vi "Acq 3.5 FPGA.vi"() -> ()   [LabVIEW 2021]
uses:
  <vilib>/rvi/Emulation/niFpgaGetClockAttributes.vi
  <vilib>/rvi/Emulation/niFpgaSctlEmulationGetInTimedLoop.vi
  <vilib>/rvi/Emulation/niFpgaEmulationReportErrorSimple.vi
  <vilib>/rvi/eio/common/nirviEmuTemplateMethod_errors.vi
  <vilib>/rvi/interface/RandomDataEmulation/niFpgaRandomDataHandleErrors.vi
  <vilib>/rvi/Emulation/niFpgaCriticalErrorInLSC.vi
  <vilib>/eio/EIONode/EIONode.xnode
  <vilib>/rvi/DataTransferAndStorage/Container/XNode/niFpgaContainer.xnode
  <vilib>/rvi/interface/RandomDataEmulation/nirviRandomDataFpgaReadWriteTemplate.vi
panel:
  in  "stop":bool
  out "CounterC/AIO":u32
  out "Acq Time (us)":u32
  in  "Count(uSec)":u32=100
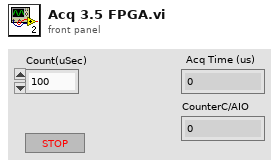
[diagram p1: front panel]
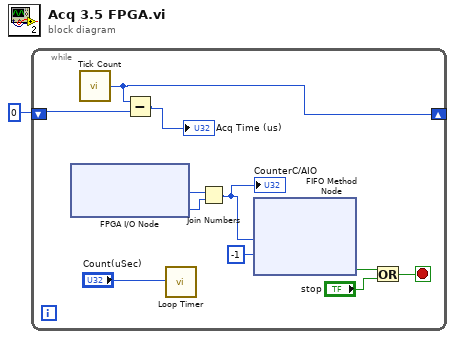
[diagram p0: block diagram]
diagram:
  n1 = while {
    shift-right: [w10] -> _
    shift-left: u32 0 -> [w12]
    stop <- w2 stop-if-true
    n2 = xnode "FPGA I/O Node"() -> ("AudioIn/Left"=w9:i16, "AudioIn/Right"=w8:i16)  [unwired: 2 in, 2 out]
    n3 = call "Tick Count"() -> ("Tick Count(uSec)"=w10:u32)
    n4 = Subtract(x=w10, y=w12) -> (x-y=→"Acq Time (us)":u32)
    n5 = call "Loop Timer"("Count(uSec)"="Count(uSec)") -> ()  [unwired: 1 out]
    n6 = Join Numbers(hi=w9, lo=w8) -> ((hi.lo)=w5:u32)
    "CounterC/AIO" <- w5
    n7 = xnode ("FIFO Method Node")("Element"=w5, "Timeout"=-1) -> ("Timed Out?"=w4:bool)  [unwired: 1 in, 1 out]
    n8 = Or(x=w4, y="stop") -> (x .or. y?=w2:bool)
  }
